vi "2022-CheesyDriveUpdated.vi"(0 "Throttle":dbl(slide)=0.007874015748031496 scale=-1.0..1.0, 1 "Custom MaxSpeedSlow (0.6)":dbl=0.6, 2 "Custom SlowRate (1)":dbl=1.0, 5 "Wheel":dbl(slide)=-0.0 scale=-1.0..1.0, 7 "Cheezy Drive Mode (2)":u16(ring)=1, 9 "CarLikeTurning":bool, 11 "Quickturn":bool, 12 "Custom MaxTurnSlow (0.55)":dbl=0.55, 13 "Custom MaxTurnRateSlow (20)":dbl=20.0) -> (4 "Left PWM":dbl, 6 "Right PWM":dbl, 10 "Selected Settings":T1)   [LabVIEW 2020]
doc: "Implements CheesyDrive. CheesyDrive means that the turn joystick controls the radius of turning instead of the rate of turning. Also implements QuickStop and QuickTurn."
panel:
  in  "FasterDeaccelerate (3)":dbl=3.0
  in  "EnableHighSensRamp (0.8)":dbl=0.8 format="%#_13g"
  in  "HighSensRamp (7)":dbl=7.0 format="%#_13g"
  in  "ArrayOfSlownesss":T2(array[cluster])=[{"MaxSpeedSlow"=1.0, "SlowRate"=5.0, "MaxTurnSlow"=1.0, "MaxTurnRateSlow"=10.0}, {"MaxSpeedSlow"=1.0, "SlowRate"=4.0, "MaxTurnSlow"=0.8, "MaxTurnRateSlow"=10.0}, {"MaxSpeedSlow"=1.0, "SlowRate"=1.0, "MaxTurnSlow"=0.55, "MaxTurnRateSlow"=10.0}, {"MaxSpeedSlow"=0.6, "SlowRate"=1.0, "MaxTurnSlow"=0.55, "MaxTurnRateSlow"=20.0}] caption="Normal\n\n\n\n\n\n\n\n\n\n\n\n\nSwitch\n\n\n\n\n\n\n\n\n\n\n\nScale\n\n\n\n\n\n\n\n\n\n\n\n\nCustom"
  in  "PointsTurn":cluster{"X":dbl, "Y":dbl}[](array[cluster])=[{"X"=0.0, "Y"=0.0}, {"X"=0.04, "Y"=0.0}, {"X"=0.041, "Y"=0.01}, {"X"=1.0, "Y"=1.0}, {"X"=1.0, "Y"=1.0}]
  in  "PointsQuickTurn":cluster{"X":dbl, "Y":dbl}[](array[cluster])=[{"X"=0.0, "Y"=0.0}, {"X"=0.04, "Y"=0.0}, {"X"=0.041, "Y"=0.2}, {"X"=0.9, "Y"=0.5}, {"X"=1.0, "Y"=1.0}]
  in  "PointsThrottle":cluster{"X":dbl, "Y":dbl}[](array[cluster])=[{"X"=0.0, "Y"=0.0}, {"X"=0.04, "Y"=0.0}, {"X"=0.0251, "Y"=0.15}, {"X"=1.0, "Y"=1.0}]
  in  "QSMult (0.1)":dbl=0.1
  in  "WheelNonLinearity (0.65)":dbl=0.65
  in  "negInertiaScalar (3)":dbl=3.0
  in  "alpha (0.1)":dbl=0.1
  out "Waveform Chart":dbl(graph)
  in  "Sensitivty (1)":dbl=1.0
  # "Enable to enable"
  # "Cheezy Drive Settings"
  # "(for quickstop decay)"
  # "Explanation:\n\"Cheesy Drive\" simply means that\n * the \"turning\" stick controls the curvature of the robot's path rather than\n * its rate of heading change. This helps make the robot more controllable at\n * high speeds. \n\nAlso handles the robot's quick turn functionality - \"quick turn\"\n * overrides constant-curvature turning for turn-in-place maneuvers.\n * Quick Stop applies backwards power to the motors to stop the robot\n * when in quick turn mode, so the robot handles better"
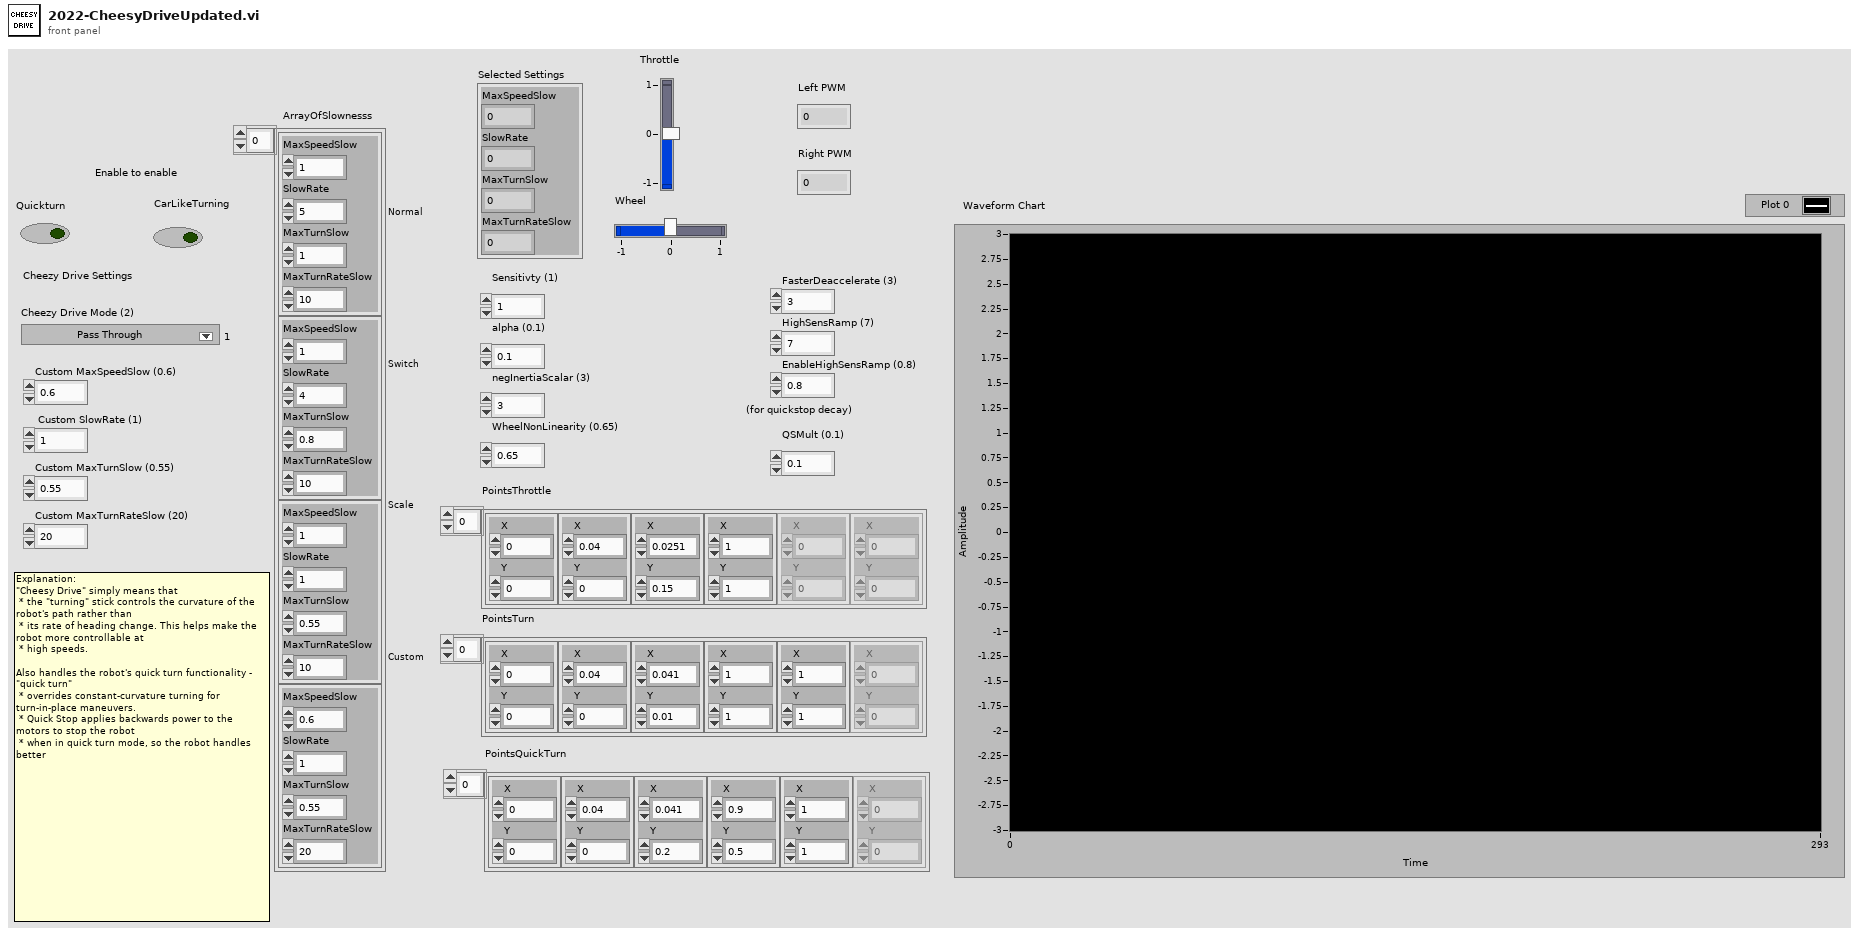
[diagram p1: front panel]
types:
  T1 = cluster{"MaxSpeedSlow":dbl, "SlowRate":dbl, "MaxTurnSlow":dbl, "MaxTurnRateSlow":dbl}
  T2 = cluster{"MaxSpeedSlow":dbl, "SlowRate":dbl, "MaxTurnSlow":dbl, "MaxTurnRateSlow":dbl}[]
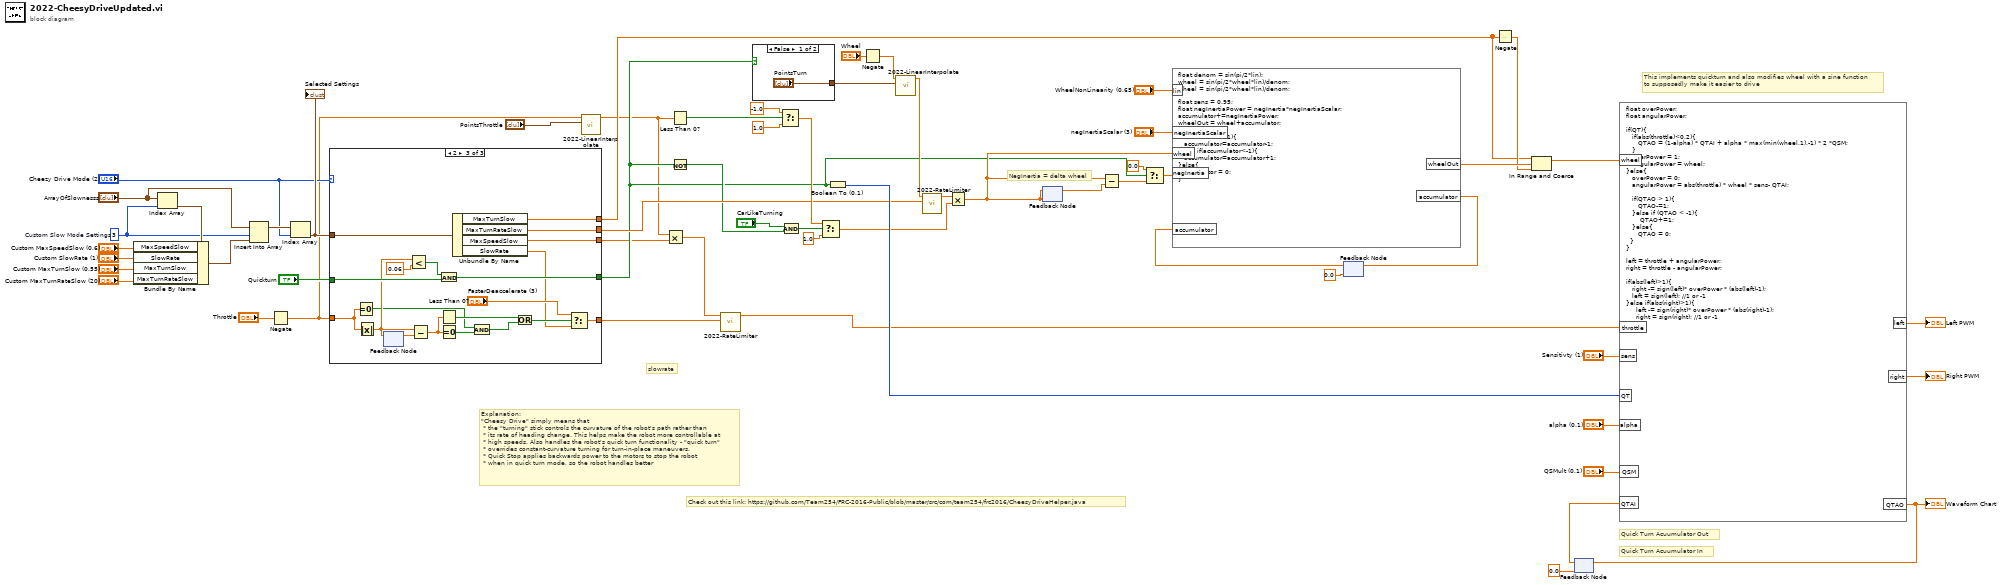
[diagram p0: block diagram]
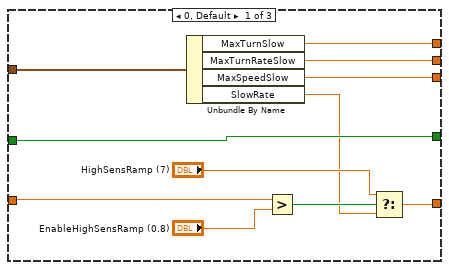
[diagram p2: hidden frame]
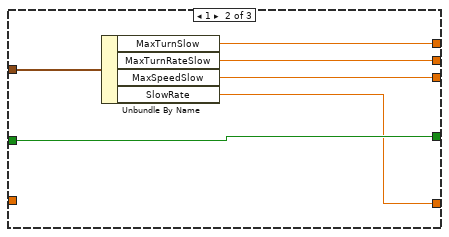
[diagram p3: hidden frame]
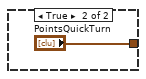
[diagram p4: hidden frame]
diagram:
  w9 = 3  # Custom Slow Mode Settings
  # "slowrate"
  # "This implements quickturn and also modifies wheel with a sine function\nto supposedly make it easier to drive"
  # "NegInertia = delta wheel"
  # "Explanation:\n\"Cheesy Drive\" simply means that\n * the \"turning\" stick controls the curvature of the robot's path rather than\n * its rate of heading change. This helps make the robot more controllable at\n * high speeds. Also handles the robot's quick turn functionality - \"quick turn\"\n * overrides constant-curvature turning for turn-in-place maneuvers.\n * Quick Stop applies backwards power to the motors to stop the robot\n * when in quick turn mode, so the robot handles better"
  # "Quick Turn Acuumulator Out"
  # "Quick Turn Acuumulator In"
  # "Check out this link: https://github.com/Team254/FRC-2016-Public/blob/master/src/com/team254/frc2016/CheesyDriveHelper.java"
  n1 = Index Array(array="ArrayOfSlownesss", index=w9) -> (element=w14:T1)
  n2 = Bundle By Name(cluster=w14, "MaxSpeedSlow"="Custom MaxSpeedSlow (0.6)", "SlowRate"="Custom SlowRate (1)", "MaxTurnSlow"="Custom MaxTurnSlow (0.55)", "MaxTurnRateSlow"="Custom MaxTurnRateSlow (20)") -> (w12:T1)
  n3 = Insert Into Array(array="ArrayOfSlownesss", index=w9, new element=w12) -> (w11:T2)
  n4 = Negate(x="Throttle") -> (-x=w2:dbl)
  n5 = Index Array(array=w11, index="Cheezy Drive Mode (2)") -> (element=w10:T1)
  "Selected Settings" <- w10
  n6 = case shown="2" "Cheezy Drive Mode (2)" {
    tunnel: [w63 w71 w88] -> w31
    tunnel: [w60 w72 w78] -> w15
    tunnel: [w68 w74 w89] -> w29
    tunnel: [w69 w75 w90] -> w26
    tunnel: "Quickturn" -> [w70 w76 w96]
    tunnel: [w70 w76 w93] -> w18
    tunnel: w2 -> [w67 _ w85]
    tunnel: w10 -> [w62 w73 w79]
    frame 0, Default {
      n7 = Unbundle By Name(w62) -> ("MaxTurnSlow"=w68:dbl, "MaxTurnRateSlow"=w69:dbl, "MaxSpeedSlow"=w60:dbl, "SlowRate"=w61:dbl)
      n8 = Greater?(x=w67, y="EnableHighSensRamp (0.8)") -> (0:w65:bool)
      n9 = Select(t="HighSensRamp (7)", s=w65, f=w61) -> (s? t:f=w63:dbl)
    }
    frame 1 {
      n10 = Unbundle By Name(w73) -> ("MaxTurnSlow"=w74:dbl, "MaxTurnRateSlow"=w75:dbl, "MaxSpeedSlow"=w72:dbl, "SlowRate"=w71:dbl)
    }
    frame 2 {
      n11 = Equal To 0?(x=w85) -> (x = 0?=w84:bool)
      n12 = Absolute Value(x=w85) -> (abs(x)=w91:dbl)
      n13 = feedback-in #1(w91) -> ()
      n14 = feedback #1() -> (w92:dbl)  [unwired: 1 in]
      n15 = Less?(x=w91, y=0.06) -> (x < y?=w95:bool)
      n16 = Subtract(x=w91, y=w92) -> (x-y=w83:dbl)
      n17 = And(x=w95, y=w96) -> (x .and. y?=w93:bool)
      n18 = Less Than 0?(x=w83) -> (x < 0?=w86:bool)
      n19 = Equal To 0?(x=w83) -> (x = 0?=w81:bool)
      n20 = Unbundle By Name(w79) -> ("MaxTurnSlow"=w89:dbl, "MaxTurnRateSlow"=w90:dbl, "MaxSpeedSlow"=w78:dbl, "SlowRate"=w77:dbl)
      n21 = And(x=w84, y=w81) -> (x .and. y?=w82:bool)
      n22 = Or(x=w86, y=w82) -> (x .or. y?=w80:bool)
      n23 = Select(t="FasterDeaccelerate (3)", s=w80, f=w77) -> (s? t:f=w88:dbl)
    }
  }
  n24 = call "2022-LinearInterpolate.vi"("Points"="PointsThrottle", "Value"=w2) -> ("Output"=w17:dbl)  [unwired: 9 in]
  n25 = Multiply(x=w17, y=w15) -> (x*y=w16:dbl)
  n26 = Less Than 0?(x=w17) -> (x < 0?=w41:bool)
  n27 = Not(x=w18) -> (.not. x?=w20:bool)
  n28 = call "2022-RateLimiter.vi"("Max dx/dt"=w31, "Input"=w16) -> ("Output"=w53:dbl)  [unwired: 9 in]
  n29 = case shown="False" w18 {
    tunnel: ["PointsTurn" "PointsQuickTurn"] -> w33
    frame False {
    }
    frame True {
    }
  }
  n30 = Select(t=-1.0, s=w41, f=1.0) -> (s? t:f=w37:dbl)
  n31 = And(x="CarLikeTurning", y=w20) -> (x .and. y?=w19:bool)
  n32 = Select(t=w37, s=w19, f=1.0) -> (s? t:f=w35:dbl)
  n33 = Boolean To (0,1)(Boolean=w18) -> (0, 1=w57:i16)
  n34 = Negate(x="Wheel") -> (-x=w1:dbl)
  n35 = call "2022-LinearInterpolate.vi"("Points"=w33, "Value"=w1) -> ("Output"=w28:dbl)  [unwired: 9 in]
  n36 = call "2022-RateLimiter.vi"("Max dx/dt"=w26, "Input"=w28) -> ("Output"=w27:dbl)  [unwired: 9 in]
  n37 = Multiply(x=w27, y=w35) -> (x*y=w38:dbl)
  n38 = feedback #2(w38) -> (w50:dbl)
  n39 = feedback-in #2(w38) -> ()
  n40 = Subtract(x=w38, y=w50) -> (x-y=w24:dbl)
  n41 = Select(t=0.0, s=w18, f=w24) -> (s? t:f=w25:dbl)
  n42 = feedback #3(0.0 ("Wheel")) -> (w49:dbl)
  n43 = formula code="float denom = sin(pi/2*lin);\nwheel = sin(pi/2*wheel*lin)/denom;\nwheel = sin(pi/2*wheel*lin)/denom;\n\nfloat sens = 0.95;\nfloat negInertiaPower = negInertia*negInertiaScalar;\naccumulator+=negInertiaPower;\nwheelOut = wheel+accumulator;\n\nif(accumulator>1){\n   accumulator=accumulator-1;\n}else if(accumulator<-1){\n   accumulator=accumulator+1;\n}else{\naccumulator = 0;\n}"("wheel"=w38, "negInertia"=w25, "accumulator"=w49, "negInertiaScalar"="negInertiaScalar (3)", "lin"="WheelNonLinearity (0.65)") -> ("accumulator"=w47:dbl, "wheelOut"=w43:dbl)
  n44 = feedback-in #3(w47) -> ()
  n45 = Negate(x=w29) -> (-x=w30:dbl)
  n46 = In Range and Coerce(upper limit=w29, x=w43, lower limit=w30) -> (coerced(x)=w44:dbl)  [unwired: 1 out]
  n47 = feedback #4(0.0 ("QTAccumulatorO")) -> (w55:dbl)
  n48 = formula code="float overPower;\nfloat angularPower;\n\nif(QT){\n   if(abs(throttle)<0.2){\n      QTAO = (1-alpha) * QTAI + alpha * max(min(wheel,1),-1) * 2 *QSM;\n   }\n   overPower = 1;\n   angularPower = wheel;\n}else{\n   overPower = 0;\n   angularPower = abs(throttle) * wheel * sens- QTAI;\n\n   if(QTAO > 1){\n      QTAO-=1;\n   }else if (QTAO < -1){\n       QTAO+=1;\n   }else{\n      QTAO = 0;\n  }\n}\n\nleft = throttle + angularPower;\nright = throttle - angularPower;\n\nif(abs(left)>1){\n   right -= sign(left)* overPower * (abs(left)-1);\n   left = sign(left); //1 or -1\n}else if(abs(right)>1){\n     left -= sign(right)* overPower * (abs(right)-1);\n     right = sign(right); //1 or -1 \n}"("wheel"=w44, "throttle"=w53, "sens"="Sensitivty (1)", "QT"=w57, "alpha"="alpha (0.1)", "QTAI"=w55, "QSM"="QSMult (0.1)") -> ("left"=→"Left PWM":dbl, "right"=→"Right PWM":dbl, "QTAO"=w58:dbl)
  "Waveform Chart" <- w58
  n49 = feedback-in #4(w58) -> ()
